vi "Verify Chan Volt Cal Test.vi"(8 "error in (no error)":errorcluster, 9 "nScale":i32, 11 "nWhichChan":i32) -> (0 "error out":errorcluster, 3 "Channel Voltage Result":dbl)   [LabVIEW 2015]
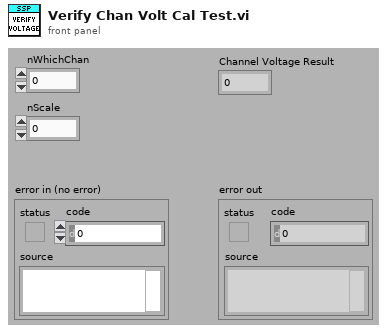
[diagram p1: front panel]
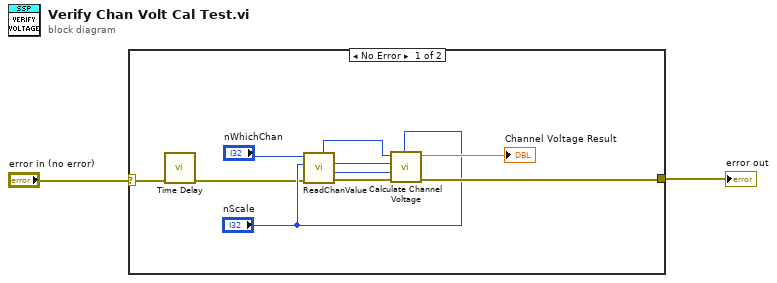
[diagram p0: block diagram]
diagram:
  n1 = case shown="No Error" "error in (no error)" {
    selector: "error in (no error)" -> [w4 w13]
    tunnel: [w7 w13] -> w2
    frame No Error {
      n2 = call "Time Delay"("error in (no error)"=w4) -> ("error out"=w3:errorcluster)  [unwired: 10 in]
      n3 = call "ReadChanValue.vi"("error in (no error)"=w3, "nScale"="nScale", "nWhichChan"="nWhichChan") -> ("error out"=w12:errorcluster, "*pnChanSpanOffset"=w9:i32, "*pnChanZeroOffset"=w10:i32, "*pnChanValue"=w11:i32)  [unwired: 4 in, 1 out]
      n4 = call "Calculate Channel Voltage.vi"("Scale"="nScale", "error in (no error)"=w12, "ChanSpanOffset"=w9, "ChanZeroOffset"=w10, "ChanValue"=w11) -> ("error out"=w7:errorcluster, "Channel Voltage Result"=→"Channel Voltage Result":dbl)  [unwired: 5 in]
    }
    frame Error {
    }
  }
  "error out" <- w2
